vi "Test coverage branch-rate 0.5 in report.vi"(11 "Test Case In":refnum<class "Coverage Report Test.lvclass">) -> (0 "error out":errorcluster, 3 "Test Case Out":refnum<class "Coverage Report Test.lvclass">)   [LabVIEW 2020, in "Coverage Report Test.lvclass"]
uses:
  Coverage Report Test.lvclass
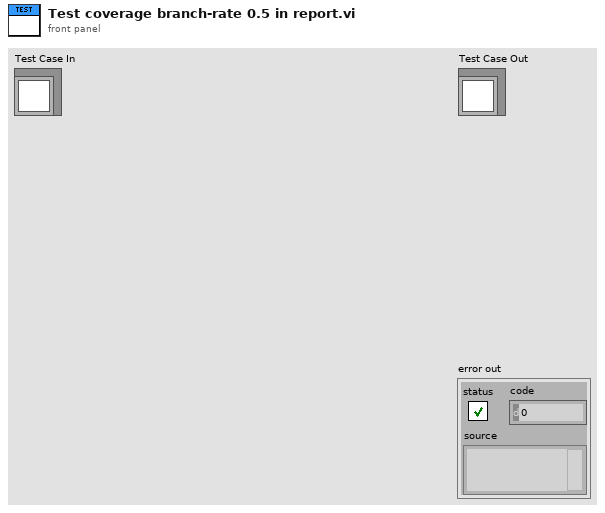
[diagram p1: front panel]
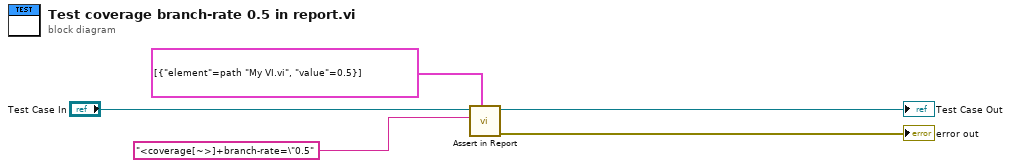
[diagram p0: block diagram]
diagram:
  n1 = call "Assert in Report.vi"("VI:s to Measure"=cluster{"element":path, "value":dbl}[] [{"element"=path "My VI.vi", "value"=0.5}], "Regular Expression"="<coverage[~>]+branch-rate=\"0.5", "Coverage Report Test in"="Test Case In") -> ("error out"=→"error out":errorcluster, "Coverage Report Test out"=→"Test Case Out":refnum<class "Coverage Report Test.lvclass">)  [unwired: 7 in]
